vi "Get Hard Disk SN.vi"(7 "当前D盘ID":u32) -> (4 "C盘ID":u32, 6 "D盘ID":u32, 8 "E盘ID":u32, 10 "F盘ID":u32, 14 "系统匹配？":bool, 15 "G盘ID":u32)   [LabVIEW 2017]
uses:
  kernel32.dll
panel:
  in  "RootPathName 5":string="g:\\"
  in  "RootPathName 4":string="f:\\"
  in  "RootPathName 3":string="e:\\"
  in  "RootPathName 2":string="d:\\"
  in  "RootPathName":string="c:\\"
  # "获取计算机盘符"
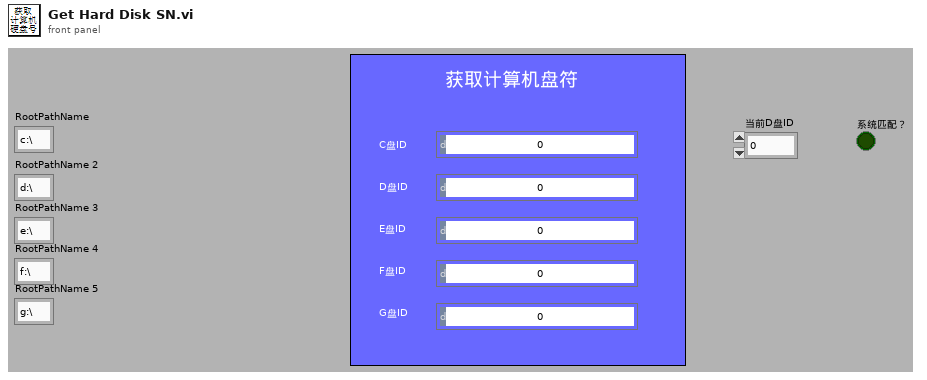
[diagram p1: front panel]
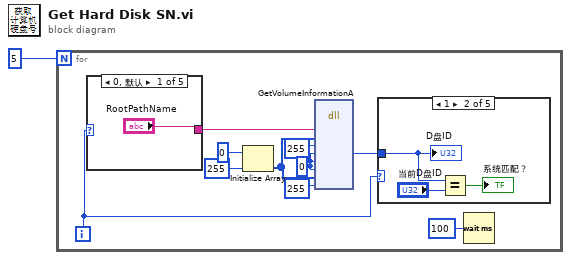
[diagram p0: block diagram]
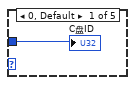
[diagram p2: hidden frame]
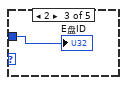
[diagram p3: hidden frame]
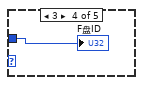
[diagram p4: hidden frame]
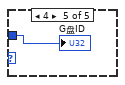
[diagram p5: hidden frame]
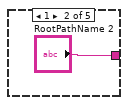
[diagram p6: hidden frame]
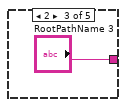
[diagram p7: hidden frame]
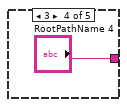
[diagram p8: hidden frame]
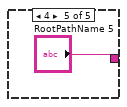
[diagram p9: hidden frame]
diagram:
  n1 = for {
    N: 5 -> [_]
    i -> [w3]
    w8 = u32 0 ("lpRootPathName")
    n2 = case shown="0, 默认" w3 {
      tunnel: ["RootPathName" "RootPathName 2" "RootPathName 3" "RootPathName 4" "RootPathName 5"] -> w6
      frame 0, Default {
      }
      frame 1 {
      }
      frame 2 {
      }
      frame 3 {
      }
      frame 4 {
      }
    }
    n3 = Initialize Array(u8 0, 255) -> (w5:u8[])
    n4 = dll-call lib="kernel32.dll" fn="GetVolumeInformationA"("lpRootPathName"=w6, "lpVolumeNameBuffer"=w5, "nVolumeNameSize"=u32 255, "lpVolumeSerialNumber"=w8, "lpMaximumComponentLength"=w8, "lpFileSystemFlags"=w8, "lpFileSystemNameBuffer"=w5, "nFileSystemNameSize"=u32 255) -> ("lpVolumeSerialNumber"=w4:u32)  [unwired: 11 in, 2 out]
    n5 = case shown="1" w3 {
      tunnel: w4 -> [w12 w15 w16 w17 w18]
      frame 0, Default {
        "C盘ID" <- w12
      }
      frame 1 {
        n6 = Equal?(x=w15, y="当前D盘ID") -> (x = y?=→"系统匹配？":bool)
        "D盘ID" <- w15
      }
      frame 2 {
        "E盘ID" <- w16
      }
      frame 3 {
        "F盘ID" <- w17
      }
      frame 4 {
        "G盘ID" <- w18
      }
    }
    n7 = Wait (ms)(milliseconds to wait=u32 100) -> ()  [unwired: 1 out]
  }
